vi "Stop Core.vi"(10 "final error code":i32, 11 "Device in":refnum<class "Device.lvclass">) -> (3 "Device out":refnum<class "Device.lvclass">)   [LabVIEW 2014, in "Device.lvclass"]
doc: "(<B>Filename</B>: Actor Framework.lvlib:Actor.lvclass:Stop Core.vi)\n\nDefines what the actor does before it stops. Use the <B>final error code</B> input to determine whether the actor shut down in response to an error.\n\nBy default, this method does nothing. A descendant class may override it to define behavior, such as shutting down any processes the actor initiated in its override of the Actor Core method."
uses:
  Device.lvclass
  Interfaces/Pipelined Actor/Pipelined Actor.lvclass
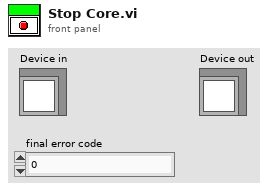
[diagram p1: front panel]
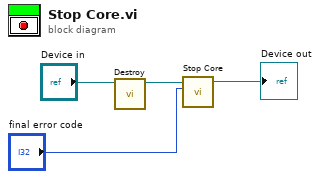
[diagram p0: block diagram]
diagram:
  n1 = call-dynamic "Destroy.vi"("Device in"="Device in") -> ("Device out"=w1:refnum<class "Device.lvclass">)  [unwired: 10 in]
  n2 = call-parent "Stop Core.vi"("final error code"="final error code", "Observable Actor in"=w1) -> ("Observable Actor out"=→"Device out":refnum<class "Device.lvclass">)  [unwired: 9 in]
